vi "DrivePath.vi"(3 "Parameter String":string, 4 "Reinit":bool) -> (0 "Path Follow Error":errorcluster, 1 "Increment":bool)   [LabVIEW 2019]
doc: "A pure-pursuit path-following algorithm configured for a swerve drive. The a feedback and a feedforward control maintain robot position while a feedback controller maintains robot orientation. This VI is designed to integrated with the FRC 4265 Autonomous Path Planner. The Search Window can be specified in seconds - longer search windows are more robust to recovering from large deviations from the path but may cause the robot to \"jump\" ahead when following tight loops or turns. The Look-Ahead Time specifies the pursuit point - this will value will directly effect the calculated positional error and the feedback-controller behavior. \n\nParameters:\n1. acceptable distance error --> (in) [0,614.25]\n2. acceptable angle error --> (deg) [0,180]\n3. path follow timeout --> (ms) [0,15000] set to -1 for no timeout\n3. name of the autonomous path"
uses:
  sensors.vi
  SafeParser_Float.vi
  SafeParser_Integer.vi
  autoninfo.vi
  dsinstructions.vi
panel:
  out "PID Distance":T1(graph)
  in  "PID Tuning Distance":T2={"Kp"=0.005, "Ki"=0.1, "Kd"=1e-08, "N-Diff"=10, "N-Int"=5, "Int Error Window"=0.5, "Max Ouput"=1.0, "Min Output"=-1.0} {"Int Error Window" min=0.0; "N-Int" min=2; "N-Diff" min=2; "Kd" min=0.0; "Ki" min=0.0; "Kp" min=0.0}
  out "PID Orientation":T1(graph)
  in  "PID Tuning Orientation":T2={"Kp"=0.01, "Ki"=0.01, "Kd"=9e-05, "N-Diff"=10, "N-Int"=10, "Int Error Window"=30.0, "Max Ouput"=1.0, "Min Output"=-1.0} {"Int Error Window" min=0.0; "N-Int" min=2; "N-Diff" min=2; "Kd" min=0.0; "Ki" min=0.0; "Kp" min=0.0}
  out "Azimuth Goal Angle":dbl(knob) scale=180.0..-180.0
  out "FF Contribution":dbl
  out "Robot Position":cluster{dbl[], dbl[]}[](graph)
  in  "Plot":bool
  in  "Look-Ahead Time (s)":dbl=0.25
  in  "Search Window (s)":dbl=2.0
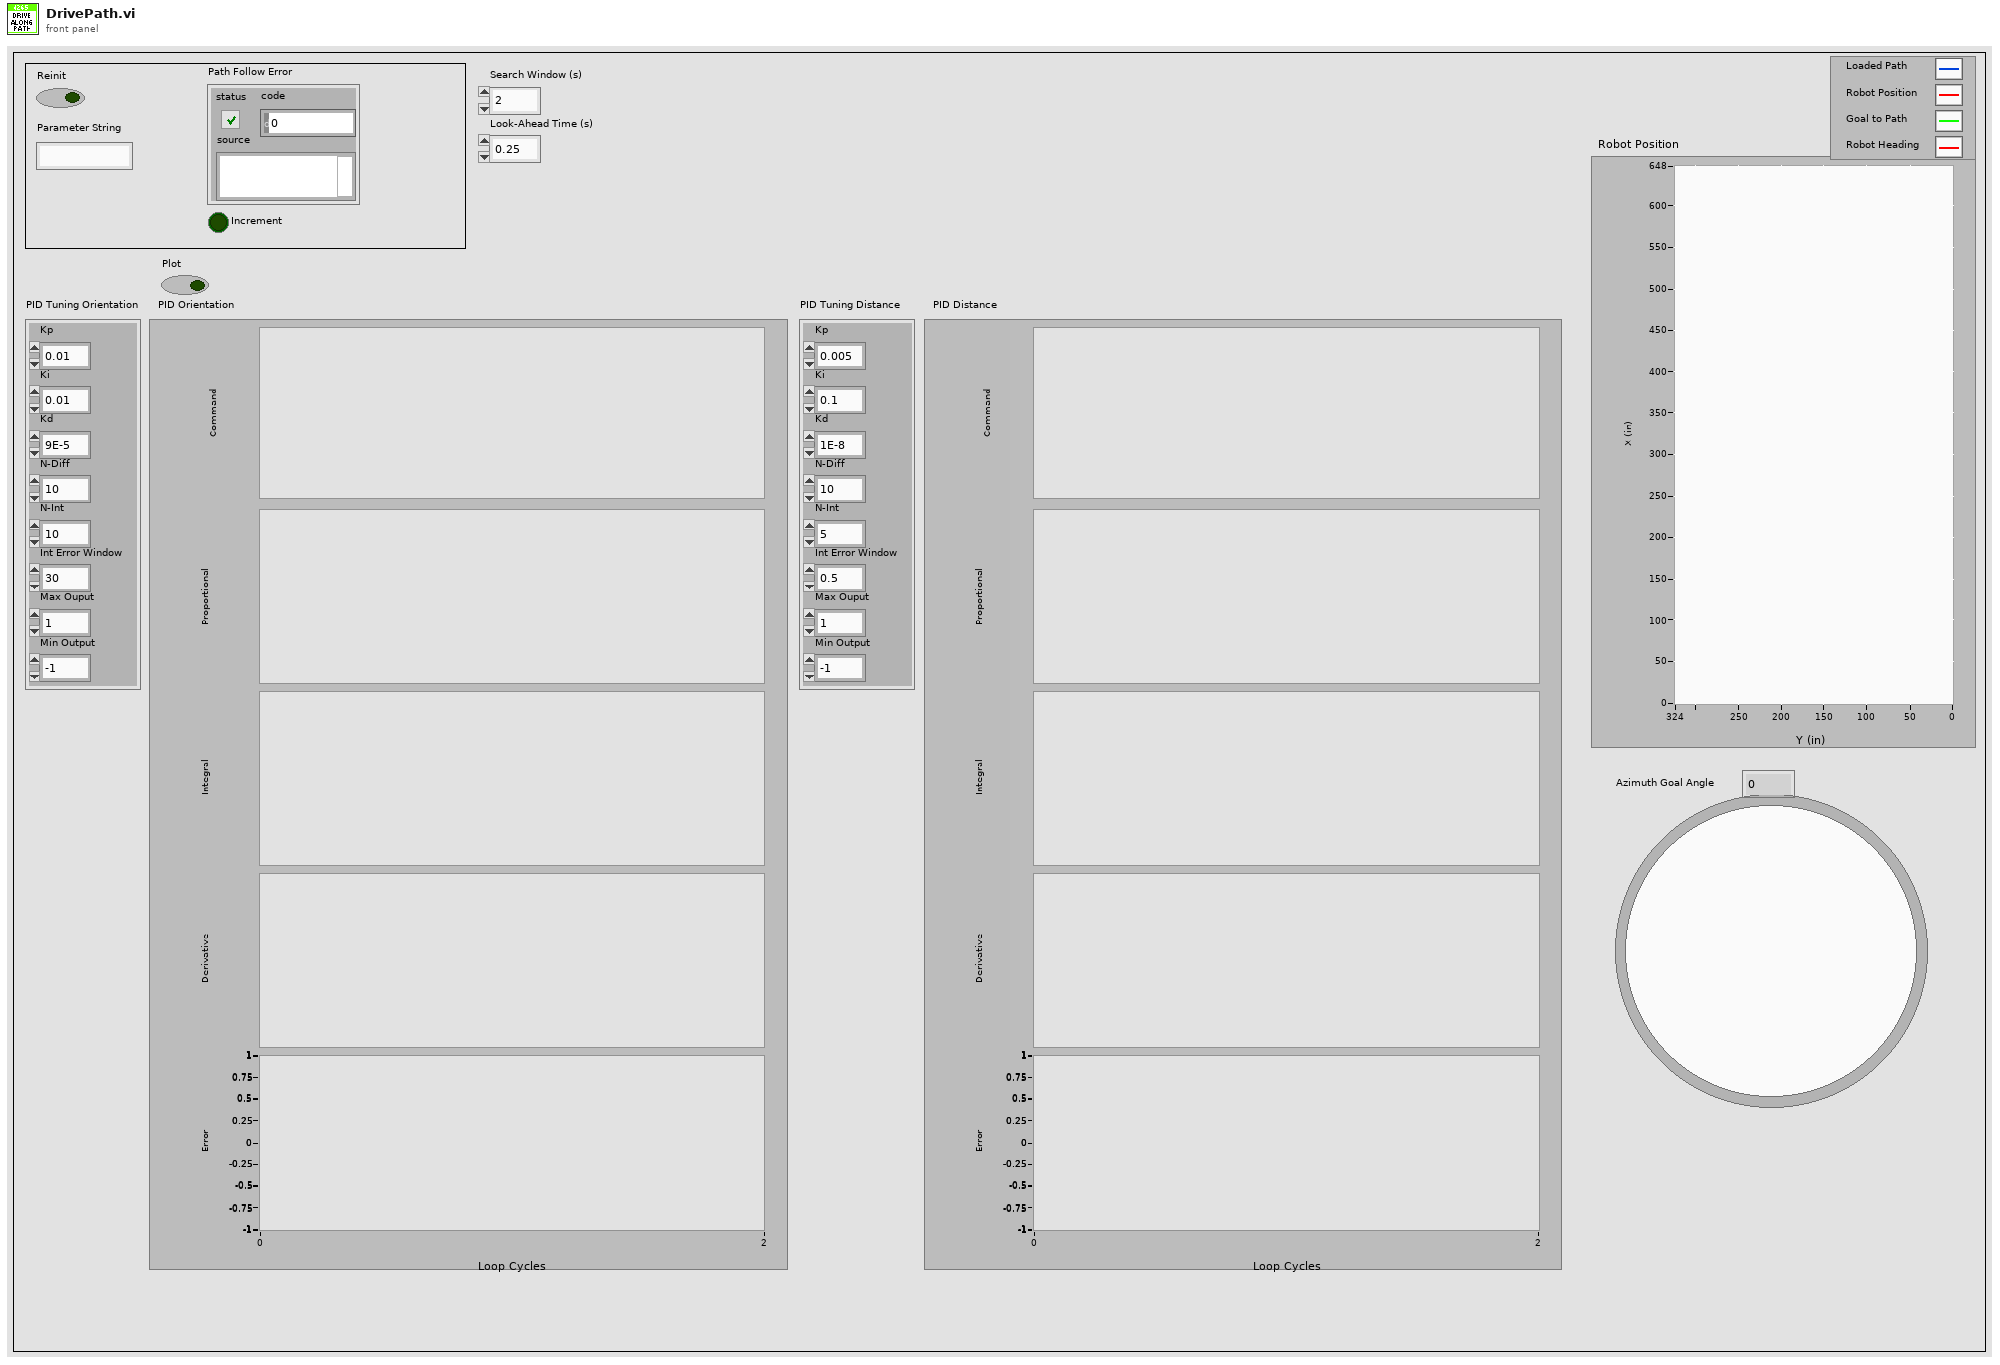
[diagram p1: front panel]
types:
  T1 = cluster{"Command":dbl, "Proportional":dbl, "Integral":dbl, "Derivative":dbl, "Goal":dbl}
  T2 = cluster{"Kp":dbl, "Ki":dbl, "Kd":dbl, "N-Diff":i32, "N-Int":i32, "Int Error Window":dbl, "Max Ouput":dbl, "Min Output":dbl}
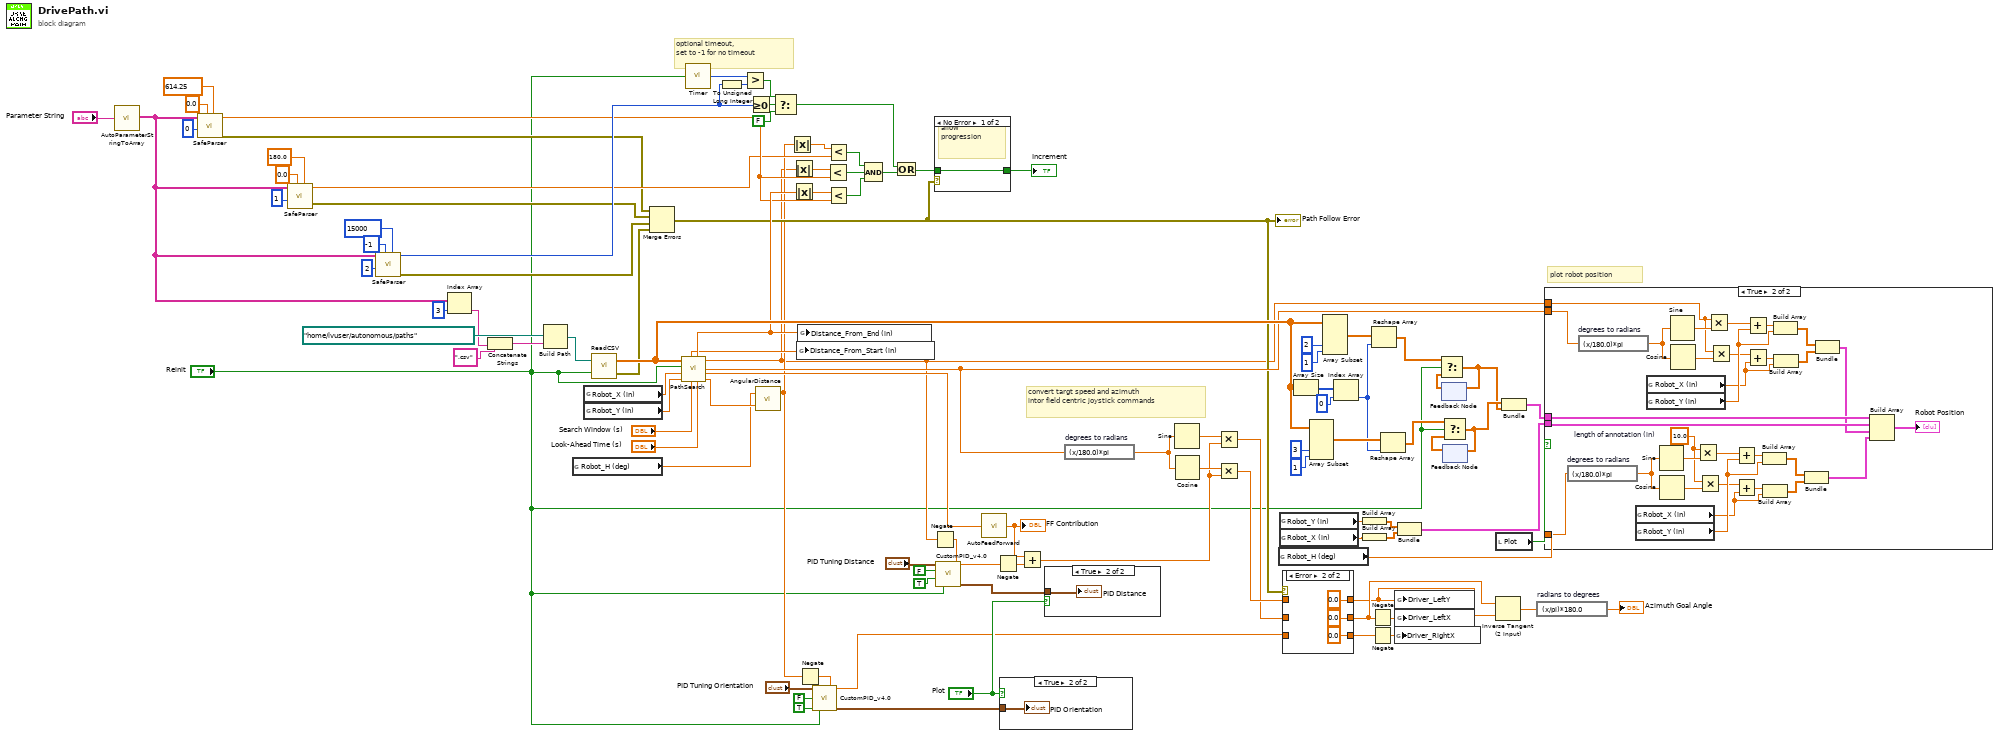
[diagram p0: block diagram]
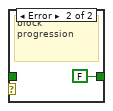
[diagram p3: hidden frame]
diagram:
  # "optional timeout,\nset to -1 for no timeout"
  # "convert targt speed and azimuth\nintor field centric joystick commands"
  # "plot robot position"
  n1 = call "AutoParameterStringToArray.vi"("Parameter String"="Parameter String") -> ("Parsed Parameters"=w26:string[])
  n2 = call-poly "SafeParser.vi"("Maximum"=614.25, "Minimum"=0.0, "Array Index"=0 ("Parameter Index"), "String Array"=w26) -> ("Error Out"=w20:errorcluster, "Typecast  Value"=w29:dbl)  [unwired: 6 in]
  n3 = call-poly "SafeParser.vi"("Maximum"=180.0, "Minimum"=0.0, "Array Index"=1 ("Parameter Index"), "String Array"=w26) -> ("Error Out"=w21:errorcluster, "Typecast  Value"=w25:dbl)  [unwired: 6 in]
  n4 = call-poly "SafeParser.vi"("Maximum"=15000, "Minimum"=-1, "Array Index"=2 ("Parameter Index"), "String Array"=w26) -> ("Error Out"=w22:errorcluster, "Typecast  Value"=w34:i32)  [unwired: 6 in]
  n5 = Index Array(array=w26, index=3) -> (element=w35:string)
  n6 = Concatenate Strings(w35, ".csv" ("string")) -> (w72:string)
  n7 = Build Path(base path=path "/home/lvuser/autonomous/paths" ("path"), name or relative path=w72) -> (appended path=w104:path)
  n8 = global read "sensors.vi" "Robot_H (deg)"() -> (w1:dbl)
  n9 = global read "sensors.vi" "Robot_X (in)"() -> (w103:dbl)
  n10 = global read "sensors.vi" "Robot_Y (in)"() -> (w102:dbl)
  n11 = call "ReadCSV.vi"("Reinit"="Reinit", "File Path (.csv)"=w104) -> ("File Open Eror"=w23:errorcluster, "Data (index by row)"=w87:dbl[][])
  n12 = Merge Errors(w20, w21, w22, w23) -> (w24:errorcluster)
  "Path Follow Error" <- w24
  n13 = call "PathSearch.vi"("Look-Ahead Time (s)"="Look-Ahead Time (s)", "Search Window (s)"="Search Window (s)", "Robot Y (in)"=w102, "Robot X (in)"=w103, "Reint"="Reinit", "Path"=w87) -> ("Angle Goal (deg)"=w38:dbl, "Velocity Goal (in/s)"=w53:dbl, "Angle To Goal (deg)"=w69:dbl, "Distance to Goal (in)"=w9:dbl, "Distance from End (in)"=w52:dbl, "Distance from Start (in)"=w51:dbl)
  n14 = call "Timer.vi"("Reset Timer"="Reinit") -> ("Time (ms)"=w39:u32)
  n15 = To Unsigned Long Integer(number=w34) -> (unsigned 32bit integer=w46:u32)
  n16 = Greater?(x=w39, y=w46) -> (0:w44:bool)
  n17 = Greater Or Equal To 0?(x=w34) -> (x >= 0?=w45:bool)
  n18 = call "AngularDistance.vi"("Goal Angle (deg) [0,360]"=w38, "Current Angle (deg) [-Inf,+Inf]"=w1) -> ("Signed Angular Distance (deg) [-180,+180]"=w16:dbl)  [unwired: 1 out]
  n19 = Select(t=w44, s=w45, f=FALSE) -> (s? t:f=w42:bool)
  n20 = Absolute Value(x=w16) -> (abs(x)=w50:dbl)
  n21 = Absolute Value(x=w9) -> (abs(x)=w41:dbl)
  n22 = Absolute Value(x=w52) -> (abs(x)=w40:dbl)
  n23 = global write "autoninfo.vi" "Distance_From_Start (in)"(w51) -> ()
  n24 = global write "autoninfo.vi" "Distance_From_End (in)"(w52) -> ()
  n25 = Negate(x=w16) -> (-x=w15:dbl)
  n26 = call "CustomPID_v4.0.vi"("PID Tuning Parameters"="PID Tuning Orientation", "Custom Error Calculation"=w15, "Reset on Goal Change ?"=FALSE, "Use Custom Error Calculation ?"=TRUE, "Reinit"="Reinit") -> ("Command"=w14:dbl, "Controller Summary"=w10:T1)  [unwired: 7 in, 2 out]
  n27 = Less?(x=w41, y=w29) -> (x < y?=w89:bool)
  n28 = Less?(x=w50, y=w25) -> (x < y?=w49:bool)
  n29 = Less?(x=w40, y=w29) -> (x < y?=w88:bool)
  n30 = Compound Arithmetic op=AND(w49, w89, w88) -> (w47:bool)
  n31 = Compound Arithmetic op=OR(w42, w47) -> (w48:bool)
  n32 = Negate(x=w9) -> (-x=w2:dbl)
  n33 = case shown="No Error" w24 {
    tunnel: [w106 FALSE] -> w74
    tunnel: w48 -> [w106 _]
    frame No Error {
      # "allow progression"
    }
    frame Error {
      # "block progression"
    }
  }
  "Increment" <- w74
  n34 = call "CustomPID_v4.0.vi"("PID Tuning Parameters"="PID Tuning Distance", "Custom Error Calculation"=w2, "Reset on Goal Change ?"=FALSE, "Use Custom Error Calculation ?"=TRUE, "Reinit"="Reinit") -> ("Command"=w3:dbl, "Controller Summary"=w7:T1)  [unwired: 7 in, 2 out]
  n35 = call "AutoFeedForward.vi"("Target Velocity (in/s)"=w53) -> ("Equivalent Joystick Command"=w54:dbl)
  "FF Contribution" <- w54
  n36 = Negate(x=w3) -> (-x=w57:dbl)
  n37 = case shown="True" "Plot" {
    tunnel: w10 -> [_ w108]
    frame False {
    }
    frame True {
      "PID Orientation" <- w108
    }
  }
  n38 = Add(x=w54, y=w57) -> (x+y=w60:dbl)
  n39 = case shown="True" "Plot" {
    tunnel: w7 -> [_ w109]
    frame False {
    }
    frame True {
      "PID Distance" <- w109
    }
  }
  n40 = expression code="(x/180.0)*pi" "degrees to radians"(w69) -> (w63:dbl)
  n41 = Sine(x=w63) -> (sin(x)=w62:dbl)
  n42 = Cosine(x=w63) -> (cos(x)=w61:dbl)
  n43 = Multiply(x=w62, y=w60) -> (x*y=w58:dbl)
  n44 = Multiply(x=w61, y=w60) -> (x*y=w59:dbl)
  n45 = global read "sensors.vi" "Robot_H (deg)"() -> (w73:dbl)
  n46 = global read "sensors.vi" "Robot_Y (in)"() -> (w86:dbl)
  n47 = global read "sensors.vi" "Robot_X (in)"() -> (w85:dbl)
  n48 = case shown="Error" w24 {
    tunnel: [w112 0.0] -> w67
    tunnel: w58 -> [w112 _]
    tunnel: [w110 0.0 ("upper limit")] -> w68
    tunnel: w59 -> [w111 _]
    tunnel: [w111 0.0] -> w66
    tunnel: w14 -> [w110 _]
    frame No Error {
    }
    frame Error {
    }
  }
  n49 = Array Size(array=w87) -> (size(s)=w92:i32[])
  n50 = Array Subset(array=w87, index (col)=3 ("index"), length (col)=1 ("length")) -> (w93:dbl[][])  [unwired: 2 in]
  n51 = Array Subset(array=w87, index (col)=2 ("index"), length (col)=1 ("length")) -> (w95:dbl[][])  [unwired: 2 in]
  n52 = Index Array(array=w92, index=0) -> (element=w90:i32)
  n53 = Build Array(w86) -> (w83:dbl[])
  n54 = Build Array(w85) -> (w84:dbl[])
  n55 = Negate(x=w67) -> (-x=w56:dbl)
  n56 = Negate(x=w68) -> (-x=w55:dbl)
  n57 = Reshape Array(w95, w90) -> (w76:dbl[])
  n58 = Reshape Array(w93, w90) -> (w94:dbl[])
  n59 = global write "dsinstructions.vi" "Driver_RightX"(w55) -> ()
  n60 = global write "dsinstructions.vi" "Driver_LeftY"(w66) -> ()
  n61 = global write "dsinstructions.vi" "Driver_LeftX"(w56) -> ()
  n62 = Bundle(w83, w84) -> (w78:cluster{dbl[], dbl[]})  [unwired: 1 in]
  n63 = feedback #1() -> (w80:dbl[])  [unwired: 1 in]
  n64 = Select(t=w76, s="Reinit", f=w80) -> (s? t:f=w81:dbl[])
  n65 = feedback-in #1(w81) -> ()
  n66 = feedback #2() -> (w79:dbl[])  [unwired: 1 in]
  n67 = Select(t=w94, s="Reinit", f=w79) -> (s? t:f=w82:dbl[])
  n68 = feedback-in #2(w82) -> ()
  n69 = local read "Plot"() -> (w75:bool)
  n70 = Inverse Tangent (2 Input)(1:w66, 2:w67) -> (0:w64:dbl)
  n71 = Bundle(w82, w81) -> (w77:cluster{dbl[], dbl[]})  [unwired: 1 in]
  n72 = expression code="(x/pi)*180.0" "radians to degrees"(w64) -> (→"Azimuth Goal Angle":dbl)
  n73 = case shown="True" w75 {
    tunnel: w78 -> [_ w145]
    tunnel: w77 -> [_ w144]
    tunnel: w9 -> [_ w132]
    tunnel: w69 -> [_ w131]
    tunnel: w73 -> [_ w118]
    frame False {
    }
    frame True {
      w117 = 10.0  # length of annotation (in)
      n74 = expression code="(x/180.0)*pi" "degrees to radians"(w118) -> (w119:dbl)
      n75 = expression code="(x/180.0)*pi" "degrees to radians"(w131) -> (w133:dbl)
      n76 = global read "sensors.vi" "Robot_X (in)"() -> (w128:dbl)
      n77 = global read "sensors.vi" "Robot_Y (in)"() -> (w129:dbl)
      n78 = global read "sensors.vi" "Robot_X (in)"() -> (w142:dbl)
      n79 = global read "sensors.vi" "Robot_Y (in)"() -> (w143:dbl)
      n80 = Sine(x=w119) -> (sin(x)=w120:dbl)
      n81 = Cosine(x=w119) -> (cos(x)=w121:dbl)
      n82 = Sine(x=w133) -> (sin(x)=w134:dbl)
      n83 = Cosine(x=w133) -> (cos(x)=w135:dbl)
      n84 = Multiply(x=w117, y=w120) -> (x*y=w122:dbl)
      n85 = Multiply(x=w117, y=w121) -> (x*y=w123:dbl)
      n86 = Multiply(x=w132, y=w134) -> (x*y=w136:dbl)
      n87 = Multiply(x=w132, y=w135) -> (x*y=w137:dbl)
      n88 = Add(x=w122, y=w129) -> (x+y=w124:dbl)
      n89 = Add(x=w123, y=w128) -> (x+y=w125:dbl)
      n90 = Add(x=w136, y=w143) -> (x+y=w138:dbl)
      n91 = Add(x=w137, y=w142) -> (x+y=w139:dbl)
      n92 = Build Array(w124, w129) -> (w126:dbl[])
      n93 = Build Array(w125, w128) -> (w127:dbl[])
      n94 = Build Array(w138, w143) -> (w140:dbl[])
      n95 = Build Array(w139, w142) -> (w141:dbl[])
      n96 = Bundle(w126, w127) -> (w116:cluster{dbl[], dbl[]})  [unwired: 1 in]
      n97 = Bundle(w140, w141) -> (w130:cluster{dbl[], dbl[]})  [unwired: 1 in]
      n98 = Build Array(w144, w145, w130, w116) -> (→"Robot Position":cluster{dbl[], dbl[]}[])
    }
  }
